vi "Get Worksheet Names.vi"(0 "Report Ref In":T1, 1 "error in (no error)":errorcluster) -> (2 "Report Ref Out":T1, 3 "Worksheet Names":string[](array[string]), 4 "error out":errorcluster)   [LabVIEW 2013, in "XCel Report Engine.lvlib"]
doc: "Returns the names of all worksheets in the open Excel report.\n\nWorksheet names are returned in workbook order. The first array element has index 0.\n\nThis VI does not change the active worksheet."
uses:
  XCel Report Engine.lvlib
  C:/Users/m.santucci/Documents/ChatGPT/LV_REPORT_ENGINE/LV/DotNet/XCelReportEngine.dll
  LV/DotNet/XCelReportEngine.dll
  Controls/Report Ref.ctl
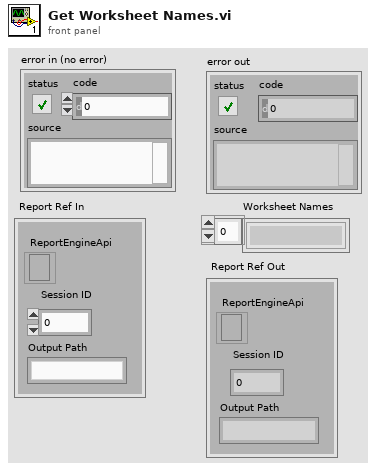
[diagram p1: front panel]
types:
  T1 = typedef "XCel Report Engine.lvlib/Report Ref.ctl" = cluster{"Session ID":i32, "Output Path":string, "ReportEngineApi":refnum<k24>}
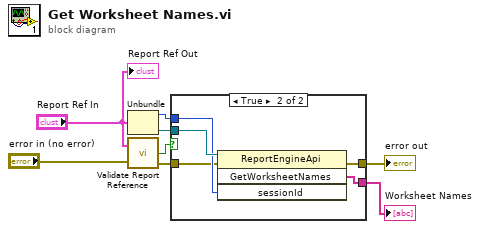
[diagram p0: block diagram]
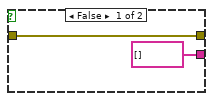
[diagram p2: hidden frame]
diagram:
  n1 = Unbundle("Report Ref In") -> ("Session ID"=w6:i32, "ReportEngineApi"=w8:refnum<k24>)  [unwired: 1 out]
  n2 = call "Validate Report Reference.vi"("Report Ref In"="Report Ref In", "error in (no error)"="error in (no error)") -> ("Valid"=w1:bool, "error out"=w2:errorcluster)  [unwired: 1 out]
  n3 = case shown="True" w1 {
    tunnel: w8 -> [_ w15]
    tunnel: [w10 w14] -> w7
    tunnel: w6 -> [_ w13]
    tunnel: [string[] [] ("GetWorksheetNames") w12] -> w5
    tunnel: w2 -> [w10 w11]
    frame False {
    }
    frame True {
      n4 = invoke class="ReportEngineApi" method="GetWorksheetNames"(reference=w15, error in=w11, "sessionId"=w13) -> (error out=w14:errorcluster, "GetWorksheetNames"=w12:string[])  [unwired: 1 in, 2 out]
    }
  }
  "error out" <- w7
  "Worksheet Names" <- w5
  "Report Ref Out" <- "Report Ref In"
